vi "Event Msg To Self.vi"(10 "Msg":refnum<class "Msg.lvclass">, 11 "jettl Event Actor in":refnum<class "jettl Event Actor.lvclass">) -> (0 "error out":errorcluster)   [LabVIEW 2021, in "jettl.lvlib" / "jettl Event Actor.lvlib" / "jettl Event Actor.lvclass"]
uses:
  jettl Event Actor.lvclass
  Actor/Msg/Msg.lvclass
  jettl Event Actor.lvclass/jettl Event Actor.ctl
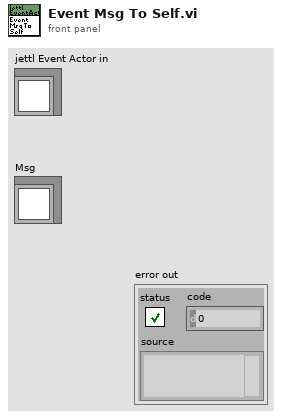
[diagram p1: front panel]
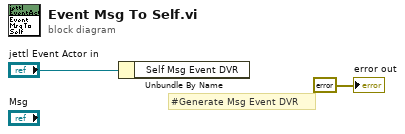
[diagram p0: block diagram]
diagram:
  # "#Generate Msg Event DVR"
  n1 = Unbundle By Name("jettl Event Actor in") -> ()  [unwired: 1 out]
  "error out" <- errorcluster {"status"=FALSE, "code"=0, "source"=""} ("error out")
